vi "Apply Objective calibration data.vi"(8 "error in (no error)":errorcluster, 10 "Current Calibration Parameters":T1 {"Slip Cycle" step=0.1; "Samples to Wait after Trigger" step=0.1; "X_norm to um_scaling" step=0.1; "Z_norm to um_scaling" step=0.1; "Distortion Correction" step=0.1; "Diff Y" step=0.1; "Diff X" step=0.1; "Sum Y" step=0.1; "Sum X" step=0.1}, 11 "Current Objective":T2="Olympus  20X") -> (0 "error out":errorcluster)   [LabVIEW 2020]
uses:
  Typedefs/Objective selector control enum.ctl
  TypeDefs/Current Calibration Parameters.ctl
  Typedefs/Calibration config.ctl
  Typedefs/Objective Config.ctl
  Typedefs/Prechirper Cal Config.ctl
  Typedefs/PreChirper constants.ctl
  Typedefs/HW config states enum.ctl
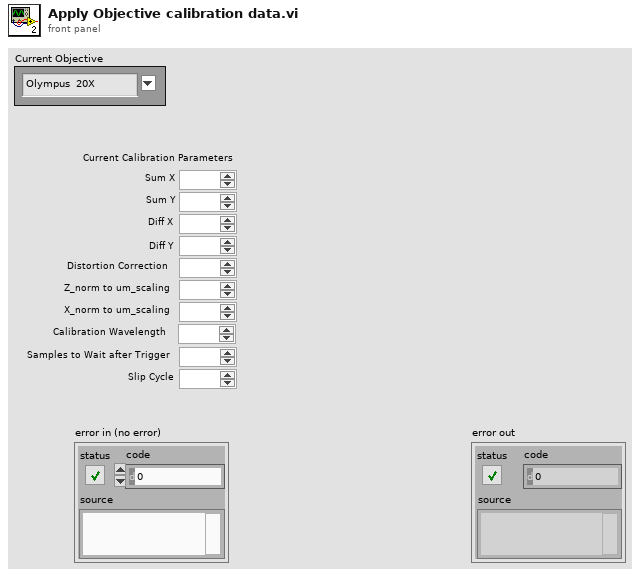
[diagram p1: front panel]
types:
  T1 = typedef "Current Calibration Parameters.ctl" = cluster{"Sum X":dbl, "Sum Y":dbl, "Diff X":dbl, "Diff Y":dbl, "Distortion Correction":dbl, "Z_norm to um_scaling":dbl, "X_norm to um_scaling":dbl, "Samples to Wait after Trigger":dbl, "Slip Cycle":dbl, "Calibration Wavelength":dbl}
  T2 = typedef "Objective selector control enum.ctl" = string
  T3 = typedef "HW config states enum.ctl" = enum16{"Load from file", "Save to file", "Save backup", "Write all", "Read all", "Write XY stage settings", "Write DAQ FPGA settings", "Write Control FPGA settings", "Write Phys Channels", "Write System Config", "Write HW Config", "Save System Config", "Save HW Config", "Clear", "Compare from file"}
  T4 = typedef "Calibration config.ctl" = cluster{"Current Objective":string, "Objective Settings":T5[], "PreChirper Values Preset ?":bool, "PreChirper Settings":T6[], "PreChirper Constants":T7}
  T5 = typedef "Objective Config.ctl" = cluster{"Name":string, "Sum X":dbl, "Sum Y":dbl, "Diff X":dbl, "Diff Y":dbl, "Distortion Correction":dbl, "Z_norm to um_scaling":dbl, "X_norm to um_scaling":dbl, "Calibrated Wavelength":dbl}
  T6 = typedef "Prechirper Cal Config.ctl" = cluster{"Wavelength":i32, "Prism 1":i32, "Prism 2":i32}
  T7 = typedef "PreChirper constants.ctl" = cluster{"a 1":i32, "b 1":i32, "c 1":i32, "a 2":i32, "b 2":i32, "c 2":i32, "lmin":i32, "lmax":i32}
  T8 = enum16{"Initialise", "Load from file", "Save to file", "Read", "Write"}
  T9 = typedef "System Configuration.ctl" = cluster{"Laser wavelength (nm)":dbl, "DAQ FPGA System":T10, "Control system":T11}
  T10 = typedef "DAQ FPGA system config.ctl" = cluster{"Clock Freq (MHz) ":dbl, "Samples Wait after Trigger":u16, "AOD fill":u16, "StartupDelay":i32, "Slip Cycle (clock cycles)":u32, "Add Cycle":bool}
  T11 = typedef "CTRL system config.ctl" = cluster{"AOD 1 Amplitude":i16, "AOD 2 Amplitude":i16, "AOD 3 Amplitude":i16, "AOD 4 Amplitude":i16, "AOD 5 Amplitude":i16, "AOD 6 Amplitude":i16, "T0 (ns)":dbl, "Ta (ns)":dbl, "Data Time Interval (ns)":dbl, "Ctrl FPGA Clock (MHz)":dbl}
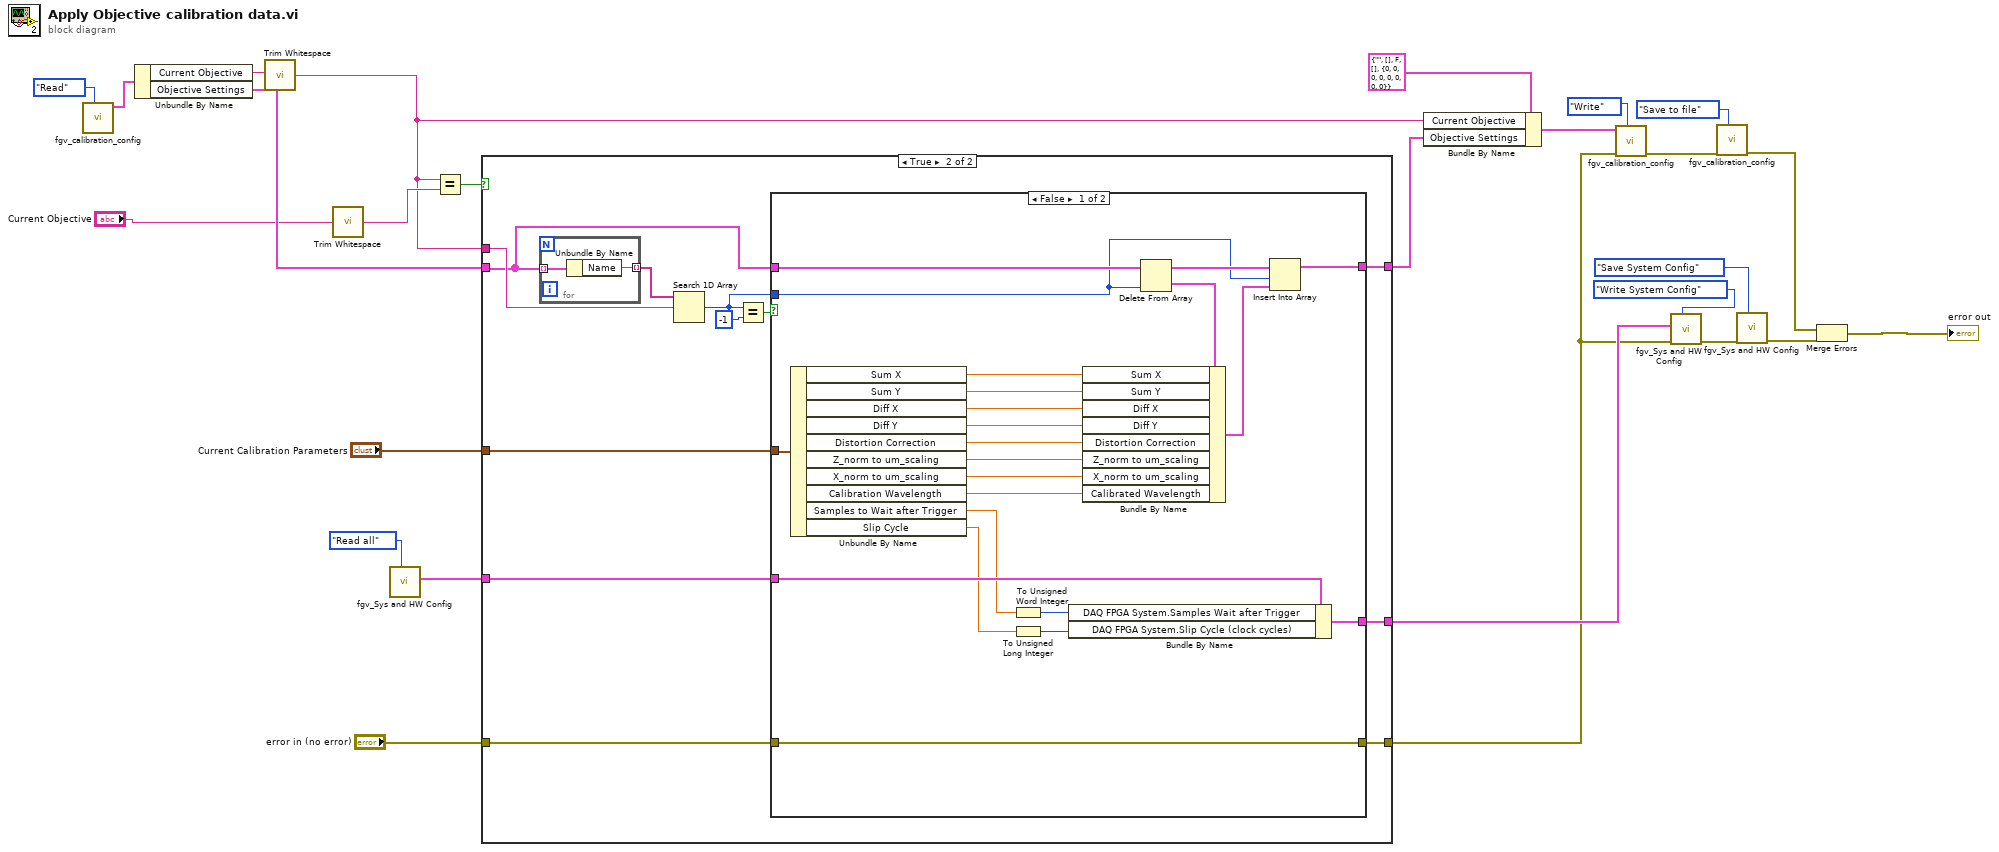
[diagram p0: block diagram]
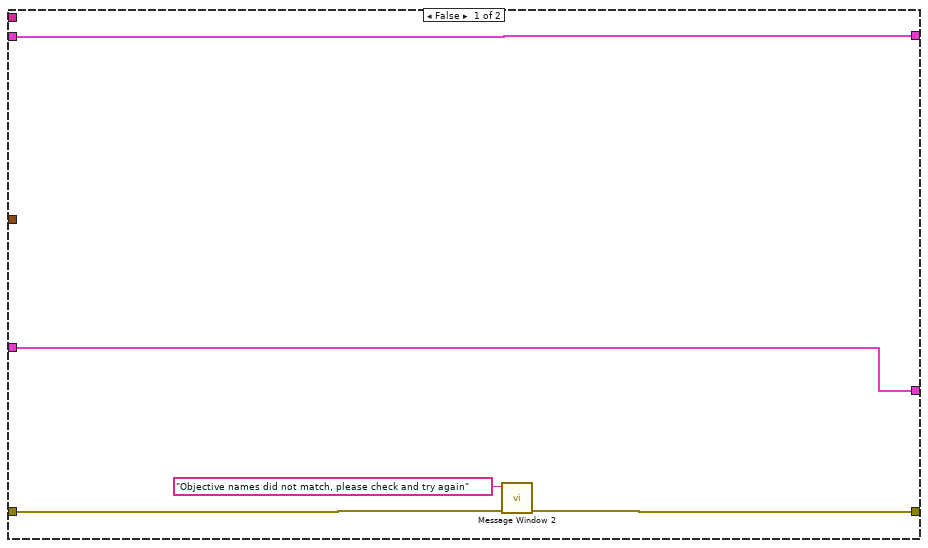
[diagram p2: hidden frame]
diagram:
  n1 = call "fgv_calibration_config.vi"("Cal config ops"=T8."Read") -> ("Config cluster OUT"=w22:T4)  [unwired: 8 in, 2 out]
  n2 = Unbundle By Name(w22) -> ("Current Objective"=w23:string, "Objective Settings"=w26:T5[])
  n3 = call <vilib>:"Trim Whitespace.vi"("string"=w23) -> ("trimmed string"=w13:string)  [unwired: 1 in]
  n4 = call <vilib>:"Trim Whitespace.vi"("string"="Current Objective") -> ("trimmed string"=w24:string)  [unwired: 1 in]
  n5 = call "fgv_Sys and HW Config.vi"("Function"=HW_config_states_enum."Read all") -> ("System Config OUT"=w8:T9)  [unwired: 8 in, 2 out]
  n6 = Equal?(x=w13, y=w24) -> (x = y?=w25:bool)
  n7 = case shown="True" w25 {
    tunnel: w26 -> [w31 w37]
    tunnel: w13 -> [_ w42]
    tunnel: [w31 w38] -> w12
    tunnel: "Current Calibration Parameters" -> [_ w36]
    tunnel: "error in (no error)" -> [w30 w35]
    tunnel: [w29 w34] -> w4
    tunnel: w8 -> [w27 w33]
    tunnel: [w27 w32] -> w7
    frame False {
      n8 = call "Message Window 2.vi"("error in (no error)"=w30, "Message string"="Objective names did not match, please check and try again") -> ("error out (no error)"=w29:errorcluster)  [unwired: 8 in, 1 out]
    }
    frame True {
      n9 = for {
        tunnel: w37 -> [w70] mode=indexing
        tunnel: [w69] -> w40 mode=indexing
        n10 = Unbundle By Name(w70) -> ("Name"=w69:string)
      }
      n11 = Search 1D Array(1D array=w40, element=w42) -> (index of element=w39:i32)  [unwired: 1 in]
      n12 = Equal?(x=w39, y=-1) -> (x = y?=w41:bool)
      n13 = case shown="False" w41 {
        tunnel: w37 -> [w65 w68]
        tunnel: w39 -> [w63 _]
        tunnel: [w62 w68] -> w38
        tunnel: w36 -> [w59 _]
        tunnel: w35 -> [w50 w67]
        tunnel: [w50 w67] -> w34
        tunnel: w33 -> [w49 w66]
        tunnel: [w44 w66] -> w32
        frame False {
          n14 = Unbundle By Name(w59) -> ("Sum X"=w58:dbl, "Sum Y"=w57:dbl, "Diff X"=w56:dbl, "Diff Y"=w55:dbl, "Distortion Correction"=w54:dbl, "Z_norm to um_scaling"=w53:dbl, "X_norm to um_scaling"=w52:dbl, "Calibration Wavelength"=w51:dbl, "Samples to Wait after Trigger"=w48:dbl, "Slip Cycle"=w45:dbl)
          n15 = To Unsigned Word Integer(number=w48) -> (unsigned 16bit integer=w47:u16)
          n16 = To Unsigned Long Integer(number=w45) -> (unsigned 32bit integer=w46:u32)
          n17 = Bundle By Name(cluster=w49, "DAQ FPGA System.Samples Wait after Trigger"=w47, "DAQ FPGA System.Slip Cycle (clock cycles)"=w46) -> (w44:T9)
          n18 = Delete From Array(array=w65, index=w63) -> (deleted portion=w61:T5, array with subset deleted=w64:T5[])  [unwired: 1 in]
          n19 = Bundle By Name(cluster=w61, "Sum X"=w58, "Sum Y"=w57, "Diff X"=w56, "Diff Y"=w55, "Distortion Correction"=w54, "Z_norm to um_scaling"=w53, "X_norm to um_scaling"=w52, "Calibrated Wavelength"=w51) -> (w60:T5)
          n20 = Insert Into Array(array=w64, index=w63, new element=w60) -> (w62:T5[])
        }
        frame True {
        }
      }
    }
  }
  n21 = Bundle By Name(cluster=T4 {"Current Objective"="", "Objective Settings"=[], "PreChirper Values Preset ?"=FALSE, "PreChirper Settings"=[], "PreChirper Constants"={"a 1"=0, "b 1"=0, "c 1"=0, "a 2"=0, "b 2"=0, "c 2"=0, "lmin"=0, "lmax"=0}} ("Config cluster IN"), "Current Objective"=w13, "Objective Settings"=w12) -> (w11:T4)
  n22 = call "fgv_calibration_config.vi"("Cal config ops"=T8."Write", "error in (no error)"=w4, "Config cluster IN"=w11) -> ("error out"=w20:errorcluster)  [unwired: 6 in, 2 out]
  n23 = call "fgv_Sys and HW Config.vi"("Function"=HW_config_states_enum."Write System Config", "error in (no error)"=w4, "System Config"=w7) -> ("error out"=w5:errorcluster)  [unwired: 6 in, 2 out]
  n24 = call "fgv_calibration_config.vi"("Cal config ops"=T8."Save to file", "error in (no error)"=w20) -> ("error out"=w2:errorcluster)  [unwired: 7 in, 2 out]
  n25 = call "fgv_Sys and HW Config.vi"("Function"=HW_config_states_enum."Save System Config", "error in (no error)"=w5) -> ("error out"=w3:errorcluster)  [unwired: 7 in, 2 out]
  n26 = Merge Errors(w2, w3) -> (→"error out":errorcluster)
